vi "set_params.vi"(8 "error in (no error)":errorcluster, 11 "glaz in":refnum<class "glaz.lvclass">) -> (0 "error out":errorcluster, 3 "glaz out":refnum<class "glaz.lvclass">)   [LabVIEW 2019, in "glaz.lvlib" / "glaz.lvclass"]
uses:
  glaz.lvclass
  C:/Users/lars/Desktop/TransientAbsorptionDAQ/_camera/_camera.lvlibp/_cameraClass/_camera.lvclass
  glaz.lvclass/glaz.ctl
  _camera/_camera.lvlibp/_cameraClass/Write wavelength.vi
panel:
  in  "driver location":path=path "C:/Program Files/National Instruments/LabVIEW 2019/user.lib/GlazLabView"
  in  "script file":path=path "C:/Users/lars/Desktop/TransientAbsorptionDAQ/cameras/glaz/no_pre_processing.gsc"
  in  "set":bool
  in  "trig delay":i32
  in  "scanCount":i32=500
  in  "internal freq":dbl=3000.0
  in  "Integration\nTime [us]":i32=2
  in  "HW Averaging":T1(ring)
  in  "Trigger Mode":enum16{"External", "Internal", "Burst"}(ring)=enum."Internal"
  in  "Integration Mode":enum16{"PulseSync", "TimeFill"}(ring)
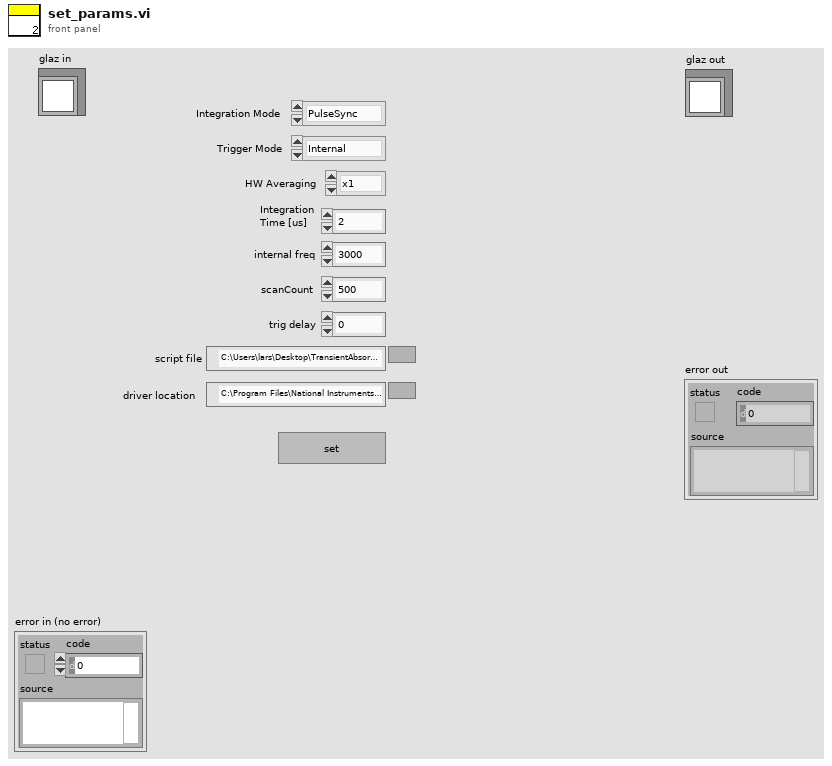
[diagram p1: front panel]
types:
  T1 = enum16{"x1", "x2", "x4", "x8", "x16", "x32", "x64", "x128", "x256"}
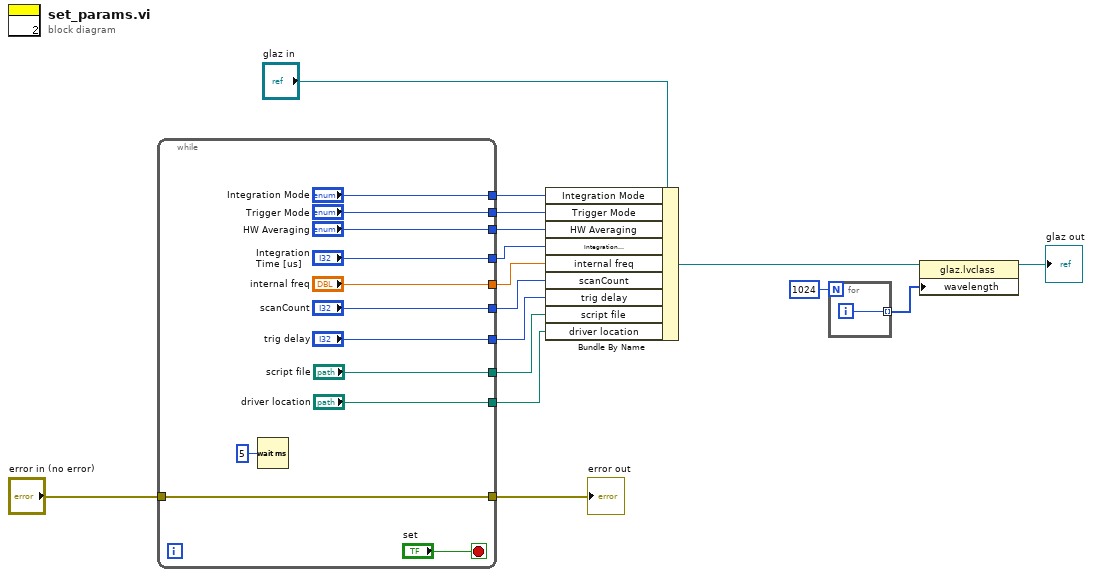
[diagram p0: block diagram]
diagram:
  n1 = while {
    tunnel: "error in (no error)" -> [w28]
    tunnel: [w28] -> w14
    tunnel: ["Integration Mode"] -> w13
    tunnel: ["Trigger Mode"] -> w12
    tunnel: ["HW Averaging"] -> w11
    tunnel: ["Integration\nTime [us]"] -> w10
    tunnel: ["internal freq"] -> w9
    tunnel: ["scanCount"] -> w8
    tunnel: ["trig delay"] -> w7
    tunnel: ["script file"] -> w6
    tunnel: ["driver location"] -> w5
    stop <- "set" stop-if-true
    n2 = Wait (ms)(milliseconds to wait=u32 5) -> ()  [unwired: 1 out]
  }
  "error out" <- w14
  n3 = Bundle By Name(cluster="glaz in", "Integration Mode"=w13, "Trigger Mode"=w12, "HW Averaging"=w11, "Integration\nTime [us]"=w10, "internal freq"=w9, "scanCount"=w8, "trig delay"=w7, "script file"=w6, "driver location"=w5) -> (w4:refnum<class "glaz.lvclass">)
  n4 = for {
    N: 1024 -> [_]
    tunnel: [w29] -> w1 mode=indexing
    i -> [w29]
  }
  n5 = property class="glaz.lvclass"(reference=w4, "wavelength"=w1) -> (reference out=→"glaz out":refnum<class "glaz.lvclass">)  [unwired: 1 in, 1 out]
